vi "subvi-simulate v1.vi"() -> (3 "Sim":bool)   [LabVIEW 2017]
uses:
  <vilib>/Platform/TimedLoop/XDataNode/timing_clust.ctl
  <vilib>/Platform/TimedLoop/XDataNode/nitl_modes.ctl
  <vilib>/Platform/TimedLoop/XDataNode/wakeup.ctl
  <vilib>/platform/TimedLoop/XDataNode/XDataNode.xnode
  <vilib>/Platform/TimedLoop/XDataNode/XDNodeRunTimeDep.lvlib
panel:
  in  "Simulate on ?":bool
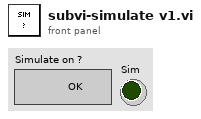
[diagram p1: front panel]
types:
  T1 = typedef "XDNodeRunTimeDep.lvlib/timing_clust.ctl" = cluster{"Expected End [f-1]":u64, "Actual End [f-1]":u64, "Finished Late? [f-1]":bool, "Expected End [i-1]":u64, "Actual End [i-1]":u64, "Finished Late? [i-1]":bool, "Expected Start [i]":u64, "Actual Start [i]":u64, "Expected Start [f]":u64, "Actual Start [f]":u64, "Source Name":string, "Structure Name":string, "Period":i64, "Deadline":i64, "Offset":i64, "Start":i64, "Priority":i32, "Timeout":i32, "Mode":T2, "Wakeup Reason":T3, "Error":errorcluster, "Source Type":string, "Secondary Source Type":string, "Global End Time":u64, "Global Start Time":u64, "Frame Duration":u64, "Iteration Duration":u64, "Assigned CPU":i32, "I/O Scan Engine Mode":u32}
  T2 = typedef "XDNodeRunTimeDep.lvlib/nitl_modes.ctl" = enum32{"No Change", "Process missed periods, maintain original phase", "Discard missed periods, maintain original phase", "Process missed periods, ignore original phase", "Discard missed periods, ignore original phase"}
  T3 = typedef "XDNodeRunTimeDep.lvlib/wakeup.ctl" = enum32{"Normal", "Aborted", "Asynchronous wakeup", "Timing source error", "Timed loop error", "Timeout"}
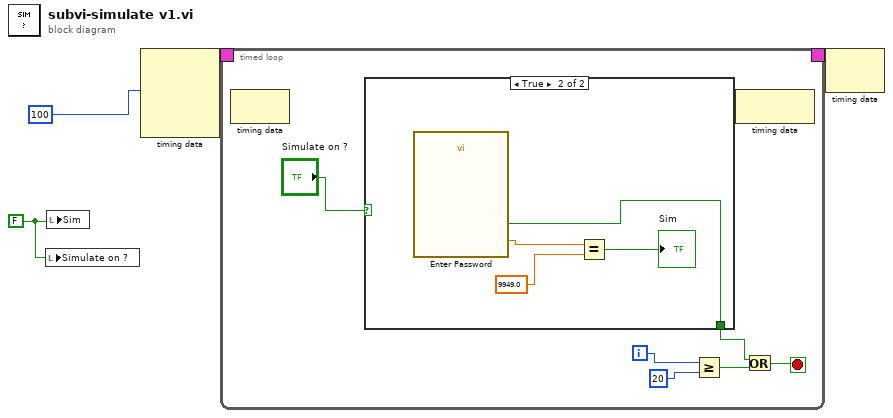
[diagram p0: block diagram]
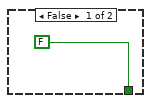
[diagram p2: hidden frame]
diagram:
  w1 = FALSE
  n1 = local write "Simulate on ?"(w1) -> ()
  n2 = local write "Sim"(w1) -> ()
  n3 = node-c288(100) -> (w4:T1)  [unwired: 3 in]
  n4 = timed-loop {
    timing: w4 -> [_]
    timing-out: [_] -> w3
    i -> [w9]
    stop <- w7 stop-if-true
    n5 = node-c288() -> ()  [unwired: 1 in, 1 out]
    n6 = case shown="True" "Simulate on ?" {
      tunnel: [FALSE w12] -> w5
      frame False {
      }
      frame True {
        n7 = call "Enter Password"() -> ("Password"=w15:dbl, "OK"=w12:bool)  [unwired: 17 in, 1 out]
        n8 = Equal?(x=w15, y=9949.0) -> (x = y?=→"Sim":bool)
      }
    }
    n9 = Greater Or Equal?(x=w9, y=20) -> (x >= y?=w6:bool)
    n10 = node-c288() -> ()  [unwired: 1 in, 1 out]
    n11 = Or(x=w5, y=w6) -> (x .or. y?=w7:bool)
  }
  n12 = node-c288(w3) -> ()  [unwired: 1 out]
